vi "Write Result of Measurement.vi"(8 "error in (no error)":errorcluster, 10 "Result Actor.lvlib:Results.lvclass":refnum<class "Results.lvclass">, 11 "Measurement in":refnum<class "Measurement.lvclass">) -> (0 "error out":errorcluster, 3 "Measurement out":refnum<class "Measurement.lvclass">)   [LabVIEW 2017, in "Measurement Actor.lvlib" / "Measurement.lvclass"]
uses:
  Measurement.lvclass
  Results/Results.lvclass
  Measurement.lvclass/Measurement.ctl
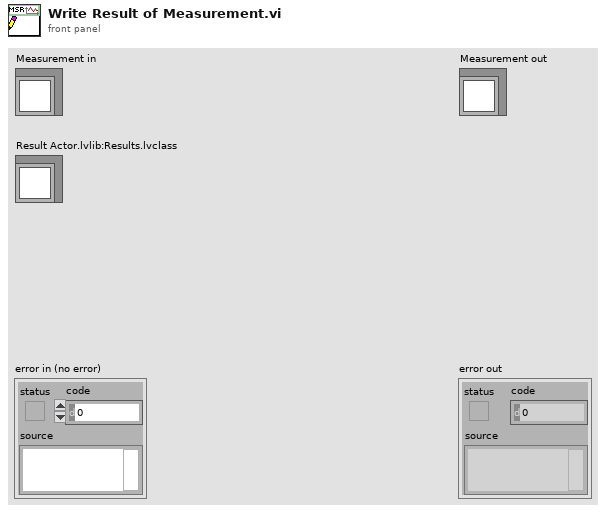
[diagram p1: front panel]
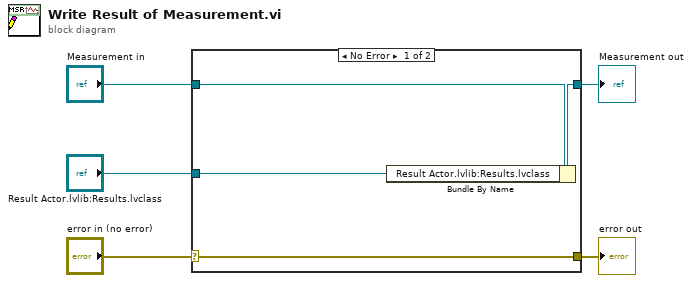
[diagram p0: block diagram]
diagram:
  n1 = case shown="No Error" "error in (no error)" {
    selector: "error in (no error)" -> [w9 w10]
    tunnel: [w9 w10] -> w4
    tunnel: [w7 w11] -> w2
    tunnel: "Measurement in" -> [w8 w11]
    tunnel: "Result Actor.lvlib:Results.lvclass" -> [w6 _]
    frame No Error {
      n2 = Bundle By Name(cluster=w8, "Result Actor.lvlib:Results.lvclass"=w6) -> (w7:refnum<class "Measurement.lvclass">)
    }
    frame Error {
    }
  }
  "error out" <- w4
  "Measurement out" <- w2
